vi "To Serial Form.vi"(6 "Serial Version":T1, 10 "Serializer in":refnum<class "Serializer.lvclass">, 11 "Single_Array in":refnum<class "Single_Array.lvclass">) -> (0 "error out":errorcluster, 2 "Serializer out":refnum<class "Serializer.lvclass">, 3 "Single_Array out":refnum<class "Single_Array.lvclass">)   [LabVIEW 2014, in "Base Data Class.lvlib" / "Single_Array.lvclass"]
uses:
  Single_Array.lvclass
  <vilib>/NI/AQ Character Lineator/Serializer/Serializer.lvclass
  <vilib>/NI/AQ Character Lineator/Serialization Common/Serial Version.ctl
  Single_Array.lvclass/Single_Array.ctl
  <vilib>/NI/AQ Character Lineator/Serializable/Insert Single Array.vi
  <vilib>/NI/AQ Character Lineator/Serializer/Insert Single Array.vi
  <vilib>/NI/AQ Character Lineator/Serializer/Read Include Default Values.vi
  Data.lvclass
  <vilib>/NI/AQ Character Lineator/Serializable/Serializable.lvclass
  <vilib>/NI/AQ Character Lineator/Serialization Common/Serialization Common.lvlib
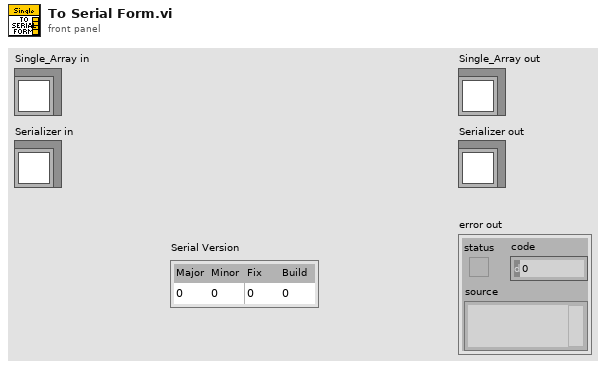
[diagram p1: front panel]
types:
  T1 = typedef "Serialization Common.lvlib/Serial Version.ctl" = cluster{"Major":u16, "Minor":u16, "Fix":u16, "Build":u16}
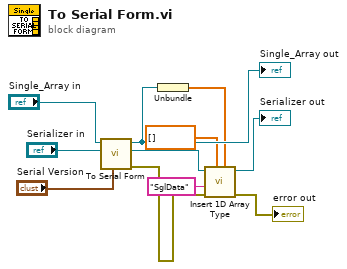
[diagram p0: block diagram]
diagram:
  n1 = call-parent "To Serial Form.vi"("Serial Version"="Serial Version", "Serializer in"="Serializer in", "Data in"="Single_Array in") -> ("error out"=w7:errorcluster, "Serializer out"=w5:refnum<class "Serializer.lvclass">, "Data out"=w8:refnum<class "Single_Array.lvclass">)  [unwired: 6 in]
  "Single_Array out" <- w8
  n2 = Unbundle(w8) -> (w6:sgl[])
  n3 = call-poly <vilib>:"Insert 1D Array Type.vi"("Singles"=w6, "Default Value"=sgl[] [], "error in (no error)"=w7, "Name"="SglData", "Serializer in"=w5) -> ("error out"=→"error out":errorcluster, "Serializer out"=→"Serializer out":refnum<class "Serializer.lvclass">)  [unwired: 5 in]
